vi "test.vi"() -> ()   [LabVIEW 2011, in "ChangeColorBtn.xctl"]
uses:
  ChangeColorBtn.xctl
panel:
  in  "可变颜色布尔按钮":bool(xcontrol)
  in  "ChangeColorBtn":bool(xcontrol)
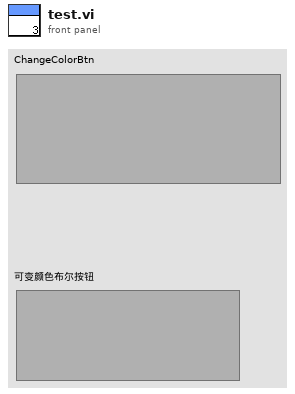
[diagram p1: front panel]
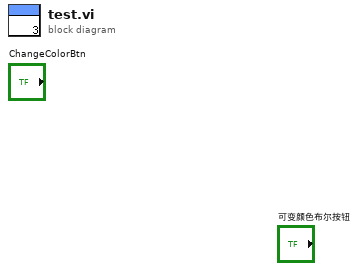
[diagram p0: block diagram]
diagram:
